vi "Myarray Reader Example.vi"() -> ()   [LabVIEW 2018]
uses:
  <vilib>/RTI DDS Toolkit/Types/RTI DDS Advanced Reader Configuration.ctl
  <vilib>/RTI DDS Toolkit/Types/RTI DDS ContentFilteredTopic Info.ctl
  <vilib>/RTI DDS Toolkit/Types/DDS Duration.ctl
  <vilib>/RTI DDS Toolkit/Types/RTI DDS Read Mode.ctl
  <vilib>/RTI DDS Toolkit/Library/LVDDS_library.lvlib
panel:
  out "Array":i64[](array[numeric])=[118, 128, 218]
  in  "LVDDS_Read_Mode":T1
  in  "Only New Samples":bool
  out "Timeout":bool
  in  "Blocking Timeout":T2
  in  "MyComplexType type":i64[](array[numeric])=[0, 0, 0]
  in  "ContentFilteredTopic Info":T3={"Filter Type"="DDS_SQLFILTER_NAME", "ContentFilteredTopic Name"="", "Filter Expression"=""}
  in  "Advanced Reader Configuration":T4={"typeName"="ros2labview_examples::msg::dds_::Intarray_", "keyName"="", "domainParticipantQoSProfile"="", "dataReaderQoSProfile"="", "forceArrayMapping?"=FALSE, "forceExclusiveReader?"=FALSE, "forceRead? (only ExclusiveReader)"=FALSE, "forceUnboundedString?"=FALSE}
  in  "error in (no error)":errorcluster
  in  "Stop Reading":bool
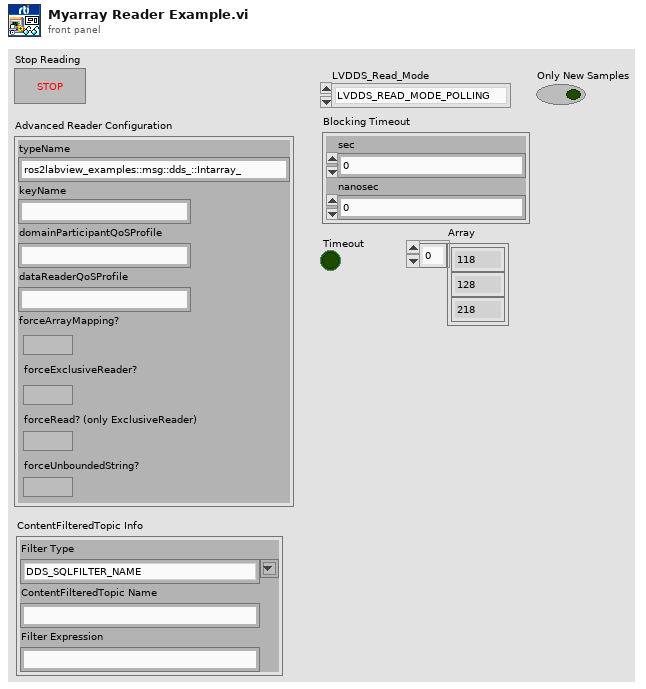
[diagram p1: front panel]
types:
  T1 = typedef "LVDDS_library.lvlib/RTI DDS Read Mode.ctl" = enum32{"LVDDS_READ_MODE_POLLING", "LVDDS_READ_MODE_BLOCKING"}
  T2 = typedef "LVDDS_library.lvlib/DDS Duration.ctl" = cluster{"sec":i32, "nanosec":u32}
  T3 = typedef "LVDDS_library.lvlib/RTI DDS ContentFilteredTopic Info.ctl" = cluster{"Filter Type":string, "ContentFilteredTopic Name":string, "Filter Expression":string}
  T4 = typedef "LVDDS_library.lvlib/RTI DDS Advanced Reader Configuration.ctl" = cluster{"typeName":string, "keyName":string, "domainParticipantQoSProfile":string, "dataReaderQoSProfile":string, "forceArrayMapping?":bool, "forceExclusiveReader?":bool, "forceRead? (only ExclusiveReader)":bool, "forceUnboundedString?":bool}
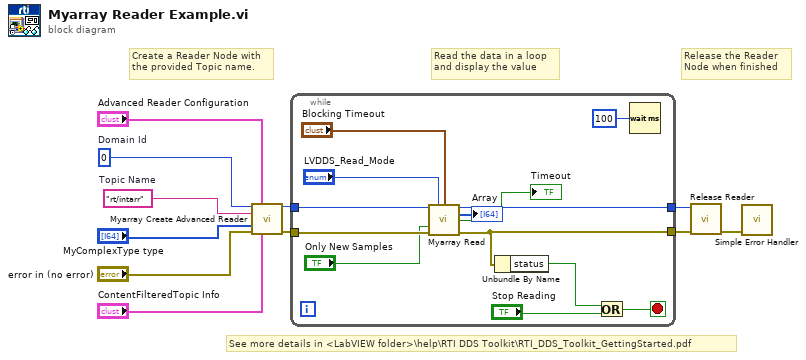
[diagram p0: block diagram]
diagram:
  w4 = "rt/intarr"  # Topic Name
  w3 = u32 0  # Domain Id
  # "See more details in <LabVIEW folder>\\help\\RTI DDS Toolkit\\RTI_DDS_Toolkit_GettingStarted.pdf"
  # "Release the Reader \nNode when finished"
  # "Read the data in a loop \nand display the value"
  # "Create a Reader Node with\nthe provided Topic name."
  n1 = call "Myarray Create Advanced Reader.vi"("Domain Id"=w3, "Advanced Reader Configuration"="Advanced Reader Configuration", "Topic Name"=w4, "MyComplexType type"="MyComplexType type", "error in (no error)"="error in (no error)", "ContentFilteredTopic Info"="ContentFilteredTopic Info") -> ("DDS Object Ref"=w8:u64, "error out"=w7:errorcluster)  [unwired: 8 in]
  n2 = while "Main Loop" {
    tunnel: w8 -> [w24]
    tunnel: [w22] -> w11
    tunnel: w7 -> [w21]
    tunnel: [w17] -> w10
    stop <- w18 stop-if-true
    n3 = call "Myarray Read.vi"("DDS Object Ref in"=w24, "Read Mode"="LVDDS_Read_Mode", "Blocking Timeout"="Blocking Timeout", "Only New Samples"="Only New Samples", "error in (no error)"=w21) -> ("DDS Object Ref out"=w22:u64, "Array"=→"Array":i64[], "Timeout"=→"Timeout":bool, "error out"=w17:errorcluster)  [unwired: 6 in, 1 out]
    n4 = Unbundle By Name(w17) -> ("status"=w20:bool)
    n5 = Or(x=w20, y="Stop Reading") -> (x .or. y?=w18:bool)
    n6 = Wait (ms)(milliseconds to wait=u32 100 ("millisecond multiple")) -> ()  [unwired: 1 out]
  }
  n7 = call <vilib>:"Release Reader.vi"("error in (no error)"=w10, "DDS Object Ref"=w11) -> ("error out"=w9:errorcluster)  [unwired: 9 in]
  n8 = call <vilib>:"Simple Error Handler.vi"("error in (no error)"=w9) -> ()  [unwired: 4 in, 5 out]
